vi "9093_第7回課題_山口修平.vi"() -> ()   [LabVIEW 2020]
panel:
  in  "START":bool
  out "電流値(A)":dbl
  out "波形チャート":dbl(graph)
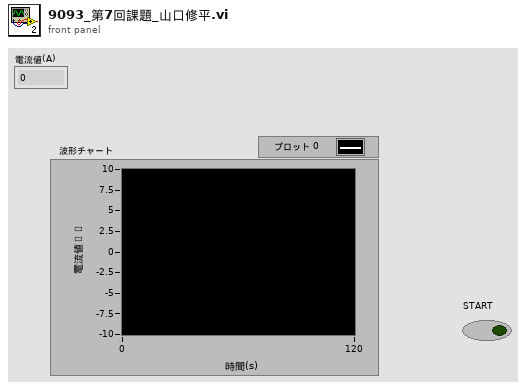
[diagram p1: front panel]
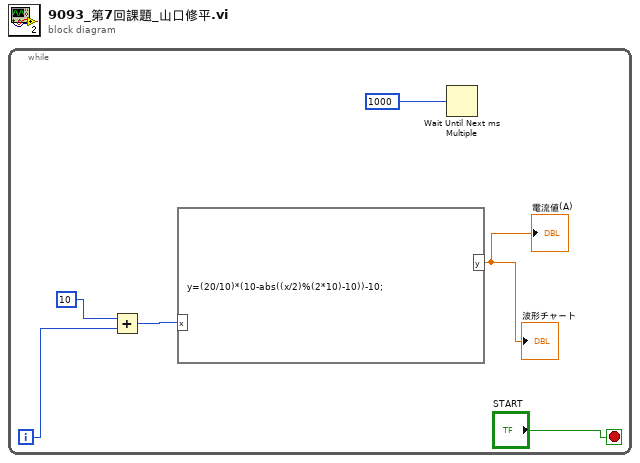
[diagram p0: block diagram]
diagram:
  n1 = while {
    i -> [w5]
    stop <- "START" stop-if-true
    n2 = Add(x=10, y=w5) -> (x+y=w4:i32)
    n3 = formula code="y=(20/10)*(10-abs((x/2)%(2*10)-10))-10;"("x"=w4) -> ("y"=→"波形チャート" →"電流値(A)":dbl)
    n4 = Wait Until Next ms Multiple(millisecond multiple=1000) -> ()  [unwired: 1 out]
  }
